vi "Set Data To Item.vi"(8 "error in (no error)":errorcluster, 11 "Tree in":refnum<class "Tree.lvclass">) -> (0 "error out":errorcluster, 3 "Tree out":refnum<class "Tree.lvclass">)   [LabVIEW 2024, in "Tree.lvclass"]
uses:
  Tree.lvclass
  Tree.lvclass/Tree.ctl
  Composite Tree Data/Composite Tree Data.lvclass
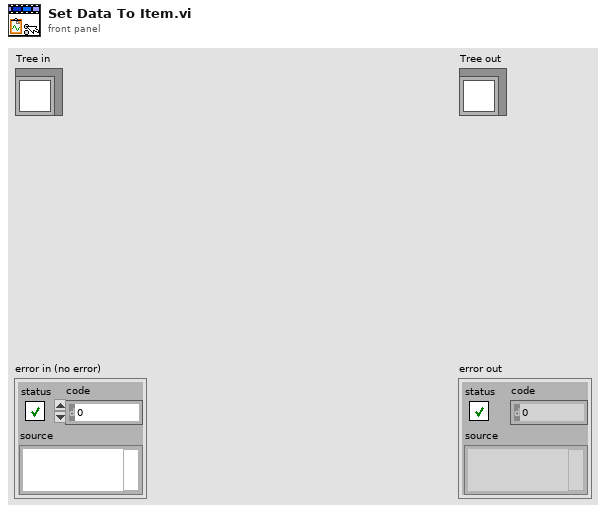
[diagram p1: front panel]
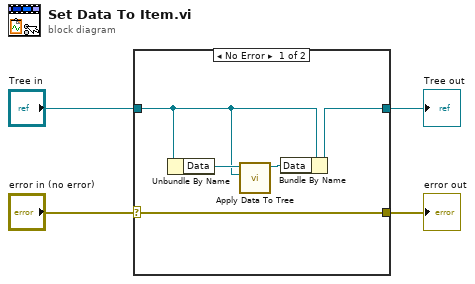
[diagram p0: block diagram]
diagram:
  n1 = case shown="No Error" "error in (no error)" {
    selector: "error in (no error)" -> [w9 w11]
    tunnel: [w9 w11] -> w3
    tunnel: [w6 w10] -> w1
    tunnel: "Tree in" -> [w5 w10]
    frame No Error {
      n2 = Unbundle By Name(w5) -> ("Data"=w8:refnum<class "Composite Tree Data.lvclass">)
      n3 = call-dynamic "Apply Data To Tree.vi"("Tree In"=w5, "Composite Tree Data in"=w8) -> ("Composite Tree Data out"=w7:refnum<class "Composite Tree Data.lvclass">)  [unwired: 7 in, 2 out]
      n4 = Bundle By Name(cluster=w5, "Data"=w7) -> (w6:refnum<class "Tree.lvclass">)
    }
    frame Error {
    }
  }
  "error out" <- w3
  "Tree out" <- w1
